vi "Display.vi"(8 "error in":errorcluster, 11 "Input (DBL) in":refnum<class "Custom - Input (DBL).lvclass">) -> (0 "error out":errorcluster, 3 "Input (DBL) out":refnum<class "Custom - Input (DBL).lvclass">)   [LabVIEW 2021, in "Pop-Up.lvlib" / "Custom - Input (DBL).lvclass"]
doc: "This vi will display the input pop up waiting for a type Double input from the user\n\nThe graphic will be an input from the developer.\n\n<b>Code Developed By:</b>\nDaniel Coons\nTechnology Service Corporation\n1983 S Liberty Drive\nBloomington, IN 47403\nPhone: 812 558-7100\ndaniel.coons@tsc.com\nwww.tsc.com/atcs"
uses:
  Custom - Input (DBL).lvclass
  C:/Development/Open Source/tsc-pop-up/Popup/Popup.lvclass
  Custom - Input (DBL).lvclass/Custom - Input (DBL).ctl
  Popup/Popup.lvclass/Popup.ctl
  Popup/Data Member Access/Read Theme.vi
  Theme/Theme.lvclass
  Popup/Popup.lvclass
  user32.dll
panel:
  out "header":bool
  in  "OK":bool
  out "Input value out":dbl=1.0 min=1.0
  out "2D Picture":picture
  out "Message":string
  in  "Input":dbl
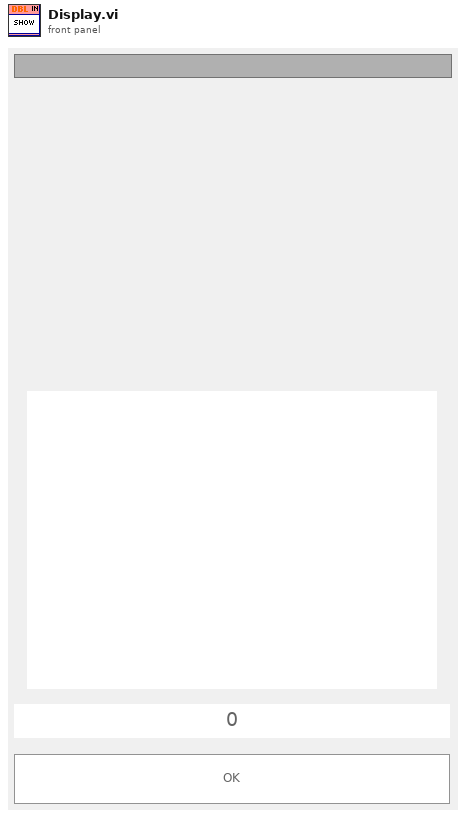
[diagram p1: front panel]
types:
  T1 = typedef "LVPoint32TypeDef.ctl" = cluster{"Horizontal":i32, "Vertical":i32}
  T2 = typedef "LVPositionTypeDef.ctl" = cluster{"Left":i32, "Top":i32}
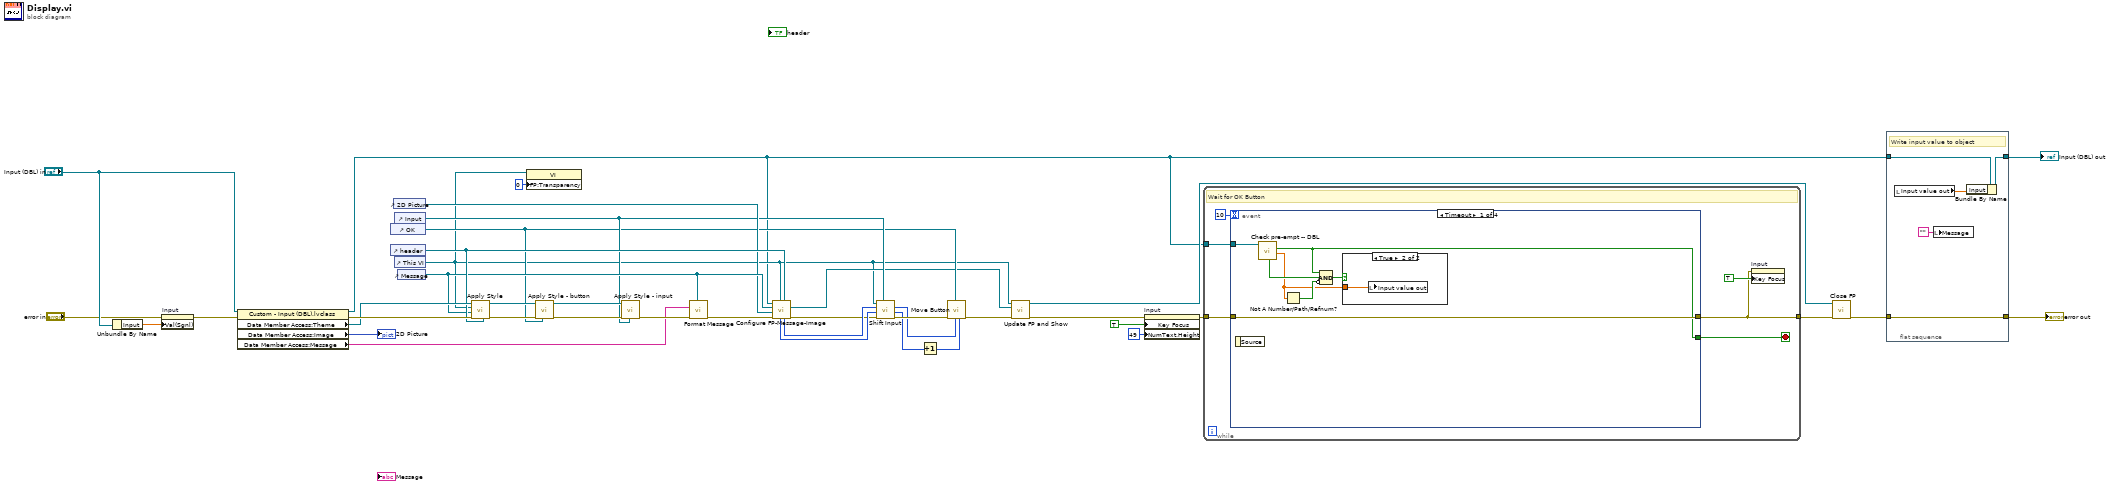
[diagram p0: block diagram]
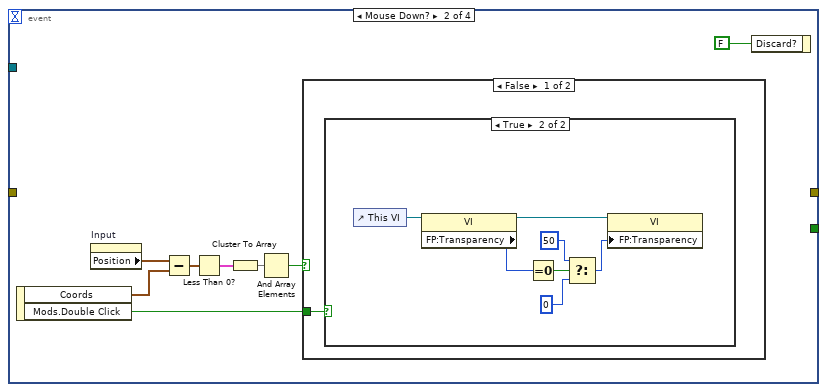
[diagram p3: hidden frame]
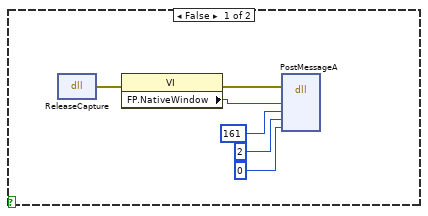
[diagram p4: hidden frame]
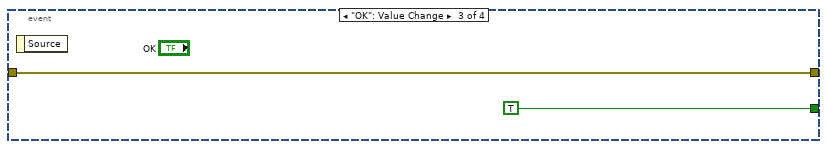
[diagram p6: hidden frame]
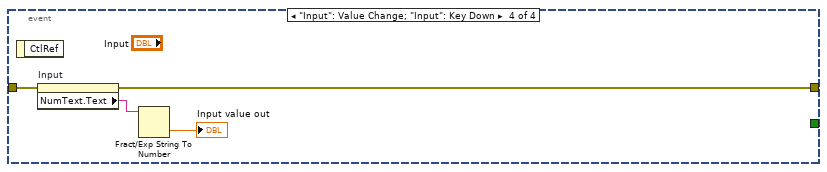
[diagram p7: hidden frame]
diagram:
  n1 = Unbundle By Name("Input (DBL) in") -> ("Input"=w35:dbl)
  n2 = property on="Input" class="DigNum (strict)"(error in="error in", "Val(Sgnl)"=w35) -> (error out=w36:errorcluster)  [unwired: 1 in, 1 out]
  n3 = property class="Custom - Input (DBL).lvclass"(reference="Input (DBL) in", error in=w36) -> (reference out=w1:refnum<class "Custom - Input (DBL).lvclass">, error out=w15:errorcluster, "Data Member Access:Theme"=w13:refnum<class "Theme.lvclass">, "Data Member Access:Image"=→"2D Picture":picture, "Data Member Access:Message"=w14:string)
  n4 = control-ref of="OK"() -> (w8:refnum<vi>)
  n5 = control-ref of="header"() -> (w12:refnum<vi>)
  n6 = control-ref of="2D Picture"() -> (w10:refnum<vi>)
  n7 = control-ref of="Input"() -> (w9:refnum<vi>)
  n8 = control-ref of="This VI"() -> (w2:refnum<vi>)
  n9 = control-ref of="Message"() -> (w11:refnum<vi>)
  n10 = call "Apply Style.vi"("header ref"=w12, "error in"=w15, "message ref"=w11, "pop up ref"=w2, "Theme in"=w13) -> ("error out"=w27:errorcluster, "Theme out"=w24:refnum<class "Theme.lvclass">)  [unwired: 5 in]
  n11 = property on="Property Node" class="VI"(reference=w2, "FP:Transparency"=u8 0 ("Front Panel Window:Transparency")) -> ()  [unwired: 1 in, 2 out]
  n12 = call "Apply Style - button.vi"("button ref"=w8, "error in"=w27, "Theme in"=w24) -> ("error out"=w26:errorcluster, "Theme out"=w23:refnum<class "Theme.lvclass">)  [unwired: 7 in]
  n13 = call "Apply Style - input.vi"("input ref"=w9, "error in (no error)"=w26, "Theme in"=w23) -> ("error out"=w25:errorcluster)  [unwired: 7 in, 1 out]
  n14 = call "Format Message.vi"("formatted string"=w11, "error in"=w25, "String Input"=w14) -> ("error out"=w28:errorcluster)  [unwired: 7 in, 1 out]
  n15 = call "Configure FP-Message-Image.vi"("header ref"=w12, "Pop Up ref"=w2, "error in (no error)"=w28, "Image ref"=w10, "Message ref"=w11, "Popup in"=w1) -> ("error out"=w17:errorcluster, "Panel Ref"=w7:refnum<vi>, "Panel Width"=w19:i32, "Panel Height"=w18:i32)  [unwired: 1 in, 1 out]
  n16 = call "Shift Input.vi"("Control"=w9, "Error In"=w17, "Panel Height"=w18, "Panel Width"=w19, "Pop Up ref"=w2) -> ("Error Out"=w22:errorcluster, "Panel Height out"=w6:i32, "Panel Width out"=w21:i32)  [unwired: 4 in]
  n17 = Increment(x=w6) -> (x+1=w20:i32)
  n18 = call "Move Button.vi"("Panel Height"=w20, "Panel Width"=w21, "Button"=w8, "Error In"=w22) -> ("Error Out"=w16:errorcluster)  [unwired: 6 in, 1 out]
  n19 = call "Update FP and Show.vi"("error in (no error)"=w16, "Panel Ref"=w7, "VI in"=w2) -> ("error out"=w32:errorcluster, "VI out"=w3:refnum<vi>)  [unwired: 7 in]
  n20 = property on="Input" class="DigNum (strict)"(error in=w32, "Key Focus"=TRUE, "NumText.Height"=u32 49 ("Numeric Text.Size:Height")) -> (error out=w31:errorcluster)  [unwired: 1 in, 1 out]
  n21 = while {
    tunnel: w1 -> [w43]
    tunnel: w31 -> [w46]
    tunnel: [w41] -> w34
    stop <- w45 stop-if-true
    # "Wait for OK Button"
    n22 = event shown="[0] Timeout" {
      selector: _ -> [_ _ _ _]
      dyn-events: _ -> [_ _ _ _]
      timeout: 10 -> [_ _ _ _]
      tunnel: w46 -> [w53 _ w78 w82]
      tunnel: [w53 _ w78 w80] -> w41
      tunnel: [w48 _ TRUE _] -> w45
      tunnel: w43 -> [w47 _ _ _]
      event Timeout {
        n23 = event-data() -> ()  [unwired: 1 in, 1 out]
        n24 = call "Check pre-empt -- DBL.vi"("_Popup in"=w47) -> ("Value?"=w49:dbl, "Pre-empted?"=w48:bool, "Type Match?"=w51:bool)  [unwired: 7 in, 1 out]
        n25 = Not A Number/Path/Refnum?(number/path/refnum=w49) -> (NaN/Path/Refnum?=w52:bool)
        n26 = Compound Arithmetic op=AND(w48, w51, invert w52) -> (w50:bool)
        n27 = case shown="True" w50 {
          tunnel: w49 -> [_ w54]
          frame False {
          }
          frame True {
            n28 = local write "Input value out"(w54) -> ()
          }
        }
      }
      event Mouse Down? {
        n29 = event-data() -> ("Coords"=w56:T1, "Mods.Double Click"=w55:bool)  [unwired: 1 in]
        n30 = property on="Input" class="DigNum (strict)"() -> ("Position"=w61:T2)  [unwired: 2 in, 2 out]
        n31 = Subtract(x=w61, y=w56) -> (x-y=w60:T2)
        n32 = Less Than 0?(x=w60) -> (x < 0?=w59:cluster{"Left":bool, "Top":bool})
        n33 = Cluster To Array(cluster=w59) -> (array=w58:bool[])
        n34 = And Array Elements(Boolean array=w58) -> (logical AND=w57:bool)
        n35 = case shown="False" w57 {
          tunnel: w55 -> [w63 _]
          frame False {
            n36 = case shown="True" w63 {
              frame False {
                n37 = dll-call lib="user32.dll" fn="ReleaseCapture"() -> (error out=w67:errorcluster)  [unwired: 4 in, 1 out]
                n38 = property class="VI"(error in=w67) -> (error out=w68:errorcluster, "FP.NativeWindow"=w69:u64)  [unwired: 1 in, 1 out]
                n39 = dll-call lib="user32.dll" fn="PostMessageA"(error in=w68, "hWnd"=w69, "Msg"=161, "wParam"=2, "lParam"=0) -> ()  [unwired: 7 in, 2 out]
              }
              frame True {
                n40 = control-ref of="This VI"() -> (w76:refnum<vi>)
                n41 = property class="VI"(reference=w76) -> (reference out=w74:refnum<vi>, "FP:Transparency"=w75:u8)  [unwired: 1 in, 1 out]
                n42 = Equal To 0?(x=w75) -> (x = 0?=w73:bool)
                n43 = Select(t=u8 50, s=w73, f=u8 0) -> (s? t:f=w72:u8)
                n44 = property class="VI"(reference=w74, "FP:Transparency"=w72) -> ()  [unwired: 1 in, 2 out]
              }
            }
          }
          frame True {
          }
        }
        n45 = event-data("Discard?"=FALSE) -> ()  [unwired: 1 in, 1 out]
      }
      event "OK": Value Change {
        n46 = event-data() -> ()  [unwired: 1 in, 1 out]
      }
      event "Input": Value Change; "Input": Key Down {
        n47 = event-data() -> ()  [unwired: 1 in, 1 out]
        n48 = property on="Input" class="DigNum (strict)"(error in=w82) -> (error out=w80:errorcluster, "NumText.Text"=w81:string)  [unwired: 1 in, 1 out]
        n49 = Fract/Exp String To Number(string=w81) -> (number=→"Input value out":dbl)  [unwired: 3 in, 1 out]
      }
    }
    n50 = property on="Input" class="DigNum (strict)"(error in=w41, "Key Focus"=TRUE) -> ()  [unwired: 1 in, 2 out]
  }
  n51 = call "Close FP.vi"("error in (no error)"=w34, "VI in"=w3) -> ("error out"=w33:errorcluster)  [unwired: 9 in]
  n52 = flat-sequence {
    tunnel: w33 -> [w87]
    tunnel: [w87] -> w37
    tunnel: w1 -> [w86]
    tunnel: [w85] -> w38
    frame #0 {
      # "Write input value to object"
      n53 = local read "Input value out"() -> (w84:dbl)
      n54 = local write "Message"("" ("Message")) -> ()
      n55 = Bundle By Name(cluster=w86, "Input"=w84) -> (w85:refnum<class "Custom - Input (DBL).lvclass">)
    }
  }
  "error out" <- w37
  "Input (DBL) out" <- w38
